vi "Test Transcriptor C2.vi"() -> ()   [LabVIEW 2014]
panel:
  in  "vi path":path=path "C:/Users/lubo/Documents/LabView/LabVIEW-Universal-Transcriptor/Test/Examples For Parsing/Blink.vi"
  out "resulting string":string
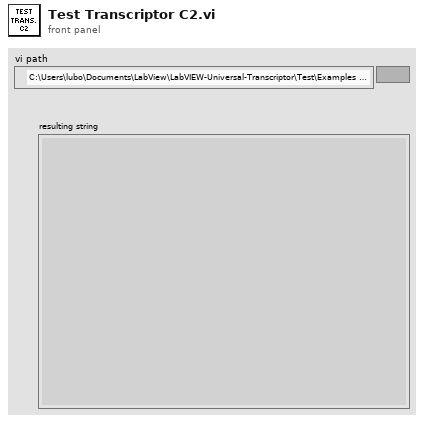
[diagram p1: front panel]
types:
  T1 = cluster{"Defines":string[], "Includes":string[], "C code":string}
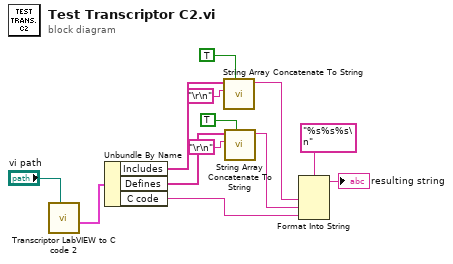
[diagram p0: block diagram]
diagram:
  n1 = call "Transcriptor LabVIEW to C code 2.vi"("vi path"="vi path") -> ("code chunks"=w13:T1)  [unwired: 7 in, 3 out]
  n2 = Unbundle By Name(w13) -> ("Includes"=w9:string[], "Defines"=w10:string[], "C code"=w5:string)
  n3 = call "String Array Concatenate To String.vi"("insert last delimiter?"=TRUE, "Delimiter char"="\r\n", "Array String In"=w9) -> ("String"=w7:string)  [unwired: 8 in]
  n4 = call "String Array Concatenate To String.vi"("insert last delimiter?"=TRUE, "Delimiter char"="\r\n", "Array String In"=w10) -> ("String"=w6:string)  [unwired: 8 in]
  n5 = Format Into String(format string="%s%s%s\n", w7, w6, w5) -> (resulting string=→"resulting string":string)  [unwired: 2 in, 1 out]
